vi "T8 Generate CPV Cmd.vi"(6 "Select CPV":i32(ring) items=["CP 24V", "CP 26V", "CP 28V", "CP 30V", "CP 31V", "CP 32V", "CP 33V", "CP 34V", "CP 35V", "CP 36V", "CP 37V", "CP 38V", "CP 39V", "CP 40V", "CP 41V", "CP 42V", "CP 43V", "CP 44V", "CP 45V", "CP 46V", "CP 47V", "CP 48V", "CP 49V", "CP 50V", "CP 51V", "CP 52V", "CP 53V", "CP 54V", "CP 56V", "CP 58V", "CP 60V", "CP 62V"], 7 "CP For Test":i32[](array[numeric]), 8 "Error In":errorcluster, 11 "Steps":i32=32) -> (0 "Error Out":errorcluster, 1 "Cmd Select":string[](array[string]), 3 "Cmd Send out":string, 4 "CP Select":i32[](array[numeric]))   [LabVIEW 2017]
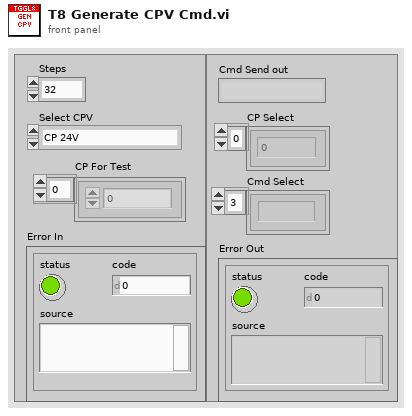
[diagram p1: front panel]
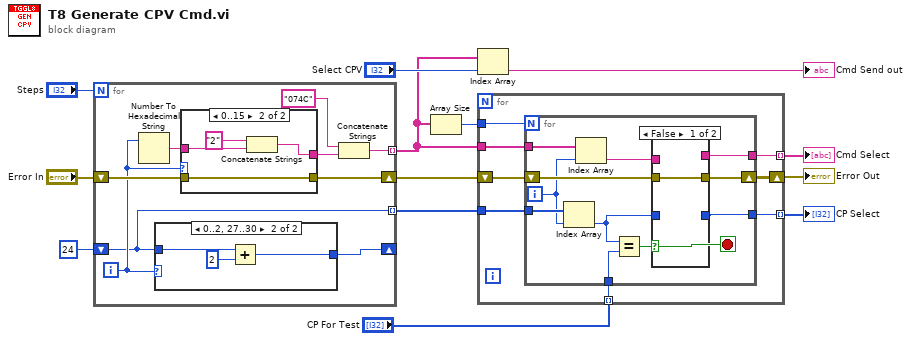
[diagram p0: block diagram]
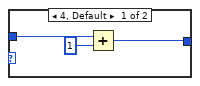
[diagram p3: hidden frame]
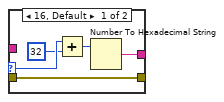
[diagram p4: hidden frame]
diagram:
  n1 = for {
    N: "Steps" -> [_]
    tunnel: [w21] -> w2 mode=indexing
    shift-right: [w17] -> w8
    shift-left: "Error In" -> [w18]
    shift-right: [w15] -> _
    shift-left: 24 -> [w14]
    tunnel: [w14] -> w6 mode=indexing
    i -> [w16]
    n2 = Number To Hexadecimal String(2:w16) -> (0:w22:string)  [unwired: 1 in]
    n3 = case shown="0..2, 27..30" w16 {
      tunnel: w14 -> [w25 w28]
      tunnel: [w23 w26] -> w15
      frame 4, Default {
        n4 = Add(x=w25, y=1) -> (x+y=w23:i32)
      }
      frame 0..2, 27..30 {
        n5 = Add(x=w28, y=2) -> (x+y=w26:i32)
      }
    }
    n6 = case shown="0..15" w16 {
      selector: w16 -> [w33 _]
      tunnel: w22 -> [_ w36]
      tunnel: [w31 w35] -> w20
      tunnel: w18 -> [w29 w34]
      tunnel: [w29 w34] -> w17
      frame 16, Default {
        n7 = Add(x=w33, y=32) -> (x+y=w32:i32)
        n8 = Number To Hexadecimal String(2:w32) -> (0:w31:string)  [unwired: 1 in]
      }
      frame 0..15 {
        n9 = Concatenate Strings("2" ("string"), w36) -> (w35:string)
      }
    }
    n10 = Concatenate Strings("074C" ("string"), w20) -> (w21:string)
  }
  n11 = Array Size(array=w2) -> (size(s)=w1:i32)
  n12 = Index Array(array=w2, index="Select CPV") -> (element=→"Cmd Send out":string)
  n13 = for {
    shift-right: [w43] -> w7
    shift-left: w8 -> [w44]
    tunnel: w2 -> [w41]
    tunnel: w6 -> [w42]
    tunnel: "CP For Test" -> [w45] mode=indexing
    tunnel: [w39] -> w4 mode=indexing
    tunnel: [w40] -> w3 mode=indexing
    tunnel: w1 -> [w38]
    n14 = for {
      N: w38 -> [_]
      tunnel: w45 -> [w56]
      shift-right: [w54] -> w43
      shift-left: w44 -> [w55]
      tunnel: w42 -> [w53]
      tunnel: w41 -> [w50]
      tunnel: [w48] -> w40
      tunnel: [w47] -> w39
      i -> [w51]
      stop <- w46 stop-if-true
      n15 = Index Array(array=w53, index=w51) -> (element=w52:i32)
      n16 = Index Array(array=w50, index=w51) -> (element=w49:string)
      n17 = Equal?(x=w52, y=w56) -> (x = y?=w46:bool)
      n18 = case shown="False" w46 {
        tunnel: w55 -> [w57 w59]
        tunnel: w49 -> [_ w60]
        tunnel: [_ w60] -> w48
        tunnel: w52 -> [_ w58]
        tunnel: [_ w58] -> w47
        tunnel: [w57 w59] -> w54
        frame False {
        }
        frame True {
        }
      }
    }
  }
  "Error Out" <- w7
  "CP Select" <- w4
  "Cmd Select" <- w3
